vi "PH_Tektronix_7000.get Channel Configuration.vi"(0 "i ref in":refnum<vi>, 1 "Channel":u16(ring) items=["Channel 1", "Channel 2", "Channel 3", "Channel 4", "Math 1", "Math 2", "Math 3", "Math 4", "Reference 1", "Reference 2", "Reference 3", "Reference 4"], 5 "error IO":errorcluster) -> (14 "i ref out":refnum<vi>, 19 "error out":errorcluster)   [LabVIEW 2014, in "PH_Tektronix_7000.lvlib"]
doc: "If the connection is established, the current channel configuration is queried and written to own attributes as well as the errors."
uses:
  PH_Tektronix_7000.lvlib
  PH_Tektronix_7000.Channel Config.ctl
  instr.lib/Tektronix7000Series/Tektronix 7000 Series - Driver np.lvlib
panel:
  in  "CH cluster":T1={"Enable Channel"=FALSE, "Bandwidth"=0, "Input Impedance"=0, "Vertical Coupling"=1, "Probe Attenuation"=1.0, "Range [V/div]"=10.0, "Position [div]"=0.0, "Bandwidth raw"=""} {"Vertical Coupling" items=["AC", "DC", "Ground"]; "Input Impedance" items=["1M", "50"]; "Bandwidth" items=["FULL", "500 MHz", "250 MHz", "150 MHz", "20 MHz"]}
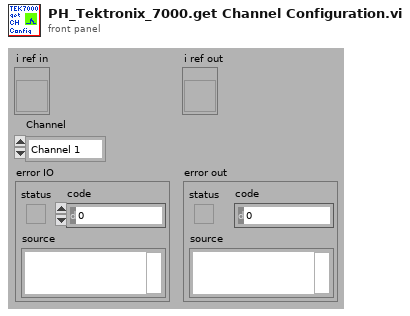
[diagram p1: front panel]
types:
  T1 = typedef "PH_Tektronix_7000.lvlib/PH_Tektronix_7000.Channel Config.ctl" = cluster{"Enable Channel":bool, "Bandwidth":u16, "Input Impedance":u16, "Vertical Coupling":u16, "Probe Attenuation":dbl, "Range [V/div]":dbl, "Position [div]":dbl, "Bandwidth raw":string}
  T2 = typedef "PH_Tektronix_7000.lvlib/PH_Tektronix_7000.i attribute.ctl" = cluster{"VISA Resource Name":refnum<visa-resource-name>, "IDN":cluster{"Instrument Driver":string, "Instrument Firmware":string, "Model":string, "Serial Number":string}, "Selftest":cluster{"Result":i32, "Message":string}, "Trigger Configuration":T3, "Acquisition Configuration":T4, "GUI Refs":T5, "State":T6, "Error Message":string, "Allow Prdc Loop?":bool, "Channel 1":T1, "Channel 2":T1, "Channel 3":T1, "Channel 4":T1, "Data CH 1":waveform(dbl), "Data CH 2":waveform(dbl), "Data CH 3":waveform(dbl), "Data CH 4":waveform(dbl), "Allow config?":bool, "Name Channel 1":string, "Name Channel 2":string, "Name Channel 3":string, "Name Channel 4":string, "Fetch Data before sending to PSDB?":bool, "Constructor passed?":bool, "Data taken at":timestamp, "Plot Colors":u32[], "Default VISA Resource":string}
  T3 = typedef "PH_Tektronix_7000.lvlib/PH_Tektronix_7000.Trigger Config.ctl" = cluster{"Source":u16, "Level [V]":dbl, "Slope":u16, "Coupling":u16, "Trigger Mode":u16}
  T4 = typedef "PH_Tektronix_7000.lvlib/PH_Tektronix_7000.Acquisition Config.ctl" = cluster{"Record Length":u32, "Timebase [s/div]":dbl, "Position [%]":dbl, "Acquisition Type":u16, "Average Waveforms":i32, "Envelope Waveforms":i32, "WfmDB Samples":i32, "Continuous?":bool, "Delay [s]":dbl, "Run?":bool}
  T5 = typedef "PH_Tektronix_7000.lvlib/PH_Tektronix_7000.GUI Refs.ctl" = cluster{"Graph":refnum<vi>, "State":refnum<vi>, "Delete":refnum<vi>, "VISA Resource":refnum<vi>, "Allow Configure":refnum<vi>, "Fetch Data":refnum<vi>, "Fetch before sending Data to PSDB":refnum<vi>, "Name Channel 1":refnum<vi>, "Name Channel 2":refnum<vi>, "Name Channel 3":refnum<vi>, "Name Channel 4":refnum<vi>, "Prdc Intervall [ms]":refnum<vi>, "Data taken":refnum<vi>, "Model":refnum<vi>, "Serial Number":refnum<vi>, "Firmware":refnum<vi>, "Driver":refnum<vi>, "Acquisition":refnum<vi>, "Trigger":refnum<vi>, "Cursor: D Time [s]":refnum<vi>, "Cursor: D Signal [V]":refnum<vi>, "Channel 1":refnum<vi>, "Channel 2":refnum<vi>, "Channel 3":refnum<vi>, "Channel 4":refnum<vi>}
  T6 = typedef "PH_StatusHandler.lvlib/PH_StatusHandler.Status.ctl" = i16
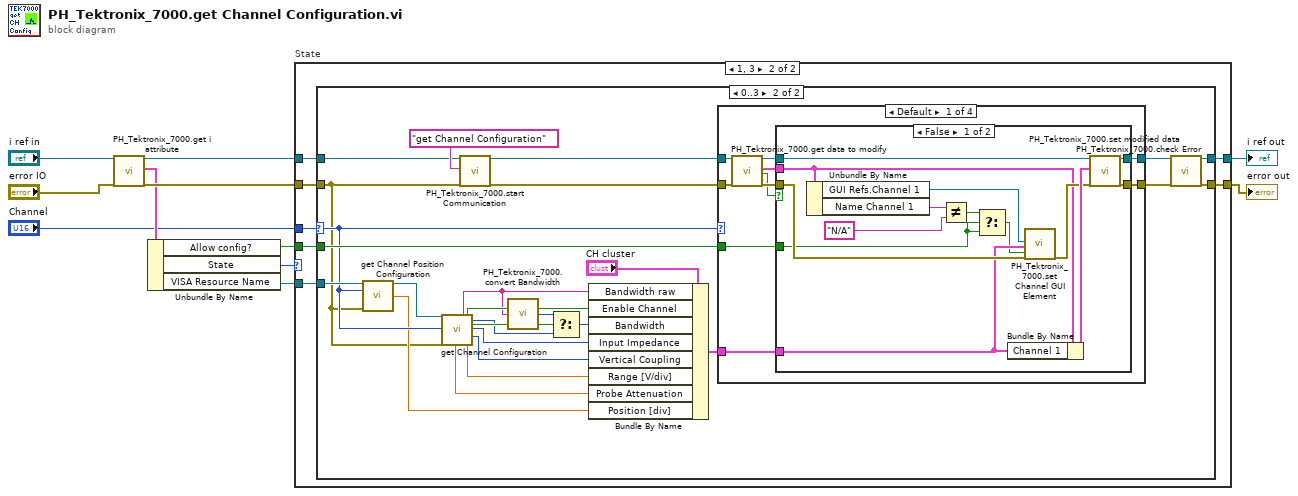
[diagram p0: block diagram]
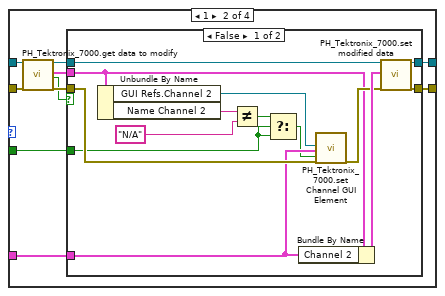
[diagram p5: hidden frame]
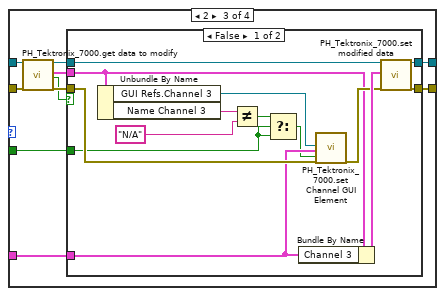
[diagram p7: hidden frame]
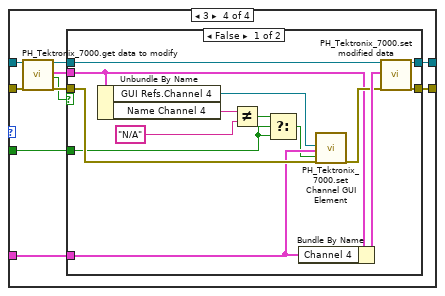
[diagram p9: hidden frame]
diagram:
  n1 = call "PH_Tektronix_7000.get i attribute.vi"("i ref in"="i ref in", "error in (no error)"="error IO") -> ("i ref out"=w7:refnum<vi>, "i attribute"=w9:T2, "error out"=w10:errorcluster)  [unwired: 15 in]
  n2 = Unbundle By Name(w9) -> ("Allow config?"=w3:bool, "State"=w2:T6, "VISA Resource Name"=w1:refnum<visa-resource-name>)
  n3 = case "State" shown="1, 3" w2 {
    tunnel: [w13 w20] -> w11
    tunnel: w10 -> [w12 w19]
    tunnel: w1 -> [_ w18]
    tunnel: w7 -> [w13 w17]
    tunnel: [w12 w16] -> w5
    tunnel: w3 -> [_ w15]
    tunnel: "Channel" -> [_ w14]
    frame Default {
    }
    frame 1, 3 {
      n4 = case shown="0..3" w14 {
        selector: w14 -> [_ w25]
        tunnel: [w22 w48] -> w20
        tunnel: w19 -> [w21 w23]
        tunnel: w18 -> [_ w38]
        tunnel: w17 -> [w22 w43]
        tunnel: [w21 w46] -> w16
        tunnel: w15 -> [_ w33]
        frame Default {
        }
        frame 0..3 {
          n5 = call "get Channel Position Configuration.vi"("VISA resource name"=w38, "Channel (0: Channel 1)"=w25, "error in (no error)"=w23) -> ("VISA resource name out"=w26:refnum<visa-resource-name>, "Vertical Position [div]"=w24:dbl)  [unwired: 10 in, 1 out]
          n6 = call "get Channel Configuration.vi"("VISA resource name"=w26, "Channel (0: Channel 1)"=w25, "error in (no error)"=w23) -> ("Probe Attenuation"=w34:dbl, "Bandwidth raw"=w28:string, "Channel enabled?"=w29:bool, "Vertical Range [V]"=w35:dbl, "Bandwidth"=w31:u16, "Bandwidth not found"=w32:bool, "Input Impedance"=w37:u16, "Vertical Coupling"=w36:u16)  [unwired: 11 in, 6 out]
          n7 = call "PH_Tektronix_7000.start Communication.vi"("i ref in"=w43, "Action"="get Channel Configuration", "error in"=w23) -> ("i ref out"=w42:refnum<vi>, "error out"=w41:errorcluster)  [unwired: 15 in]
          n8 = call "PH_Tektronix_7000.convert Bandwidth.vi"("Bandwidth raw"=w28) -> ("Bandwidth"=w27:u16)
          n9 = Select(t=w27, s=w32, f=w31) -> (s? t:f=w30:u16)
          n10 = Bundle By Name(cluster="CH cluster", "Bandwidth raw"=w28, "Enable Channel"=w29, "Bandwidth"=w30, "Input Impedance"=w37, "Vertical Coupling"=w36, "Range [V/div]"=w35, "Probe Attenuation"=w34, "Position [div]"=w24) -> (w39:T1)
          n11 = case "Channel Label" shown="Default" w25 {
            tunnel: [w54 w80 w106 w132] -> w47
            tunnel: w41 -> [w51 w77 w103 w129]
            tunnel: w42 -> [w52 w78 w104 w130]
            tunnel: [w53 w79 w105 w131] -> w45
            tunnel: w39 -> [w50 w76 w102 w128]
            tunnel: w33 -> [w49 w75 w101 w127]
            frame Default {
              n12 = call "PH_Tektronix_7000.get data to modify.vi"("i ref in"=w52, "error in (no error)"=w51) -> ("i ref out"=w57:refnum<vi>, "i attribute"=w55:T2, "timed out"=w56:bool, "error out"=w58:errorcluster)  [unwired: 14 in]
              n13 = case shown="False" w56 {
                tunnel: [w69 w73] -> w53
                tunnel: w58 -> [w68 w73]
                tunnel: w57 -> [w72 w74]
                tunnel: [w70 w74] -> w54
                tunnel: w55 -> [w66 _]
                tunnel: w50 -> [w65 _]
                tunnel: w49 -> [w63 _]
                frame False {
                  n14 = Unbundle By Name(w66) -> ("GUI Refs.Channel 1"=w59:refnum<vi>, "Name Channel 1"=w62:string)
                  n15 = Not Equal?(x=w62, y="N/A") -> (x != y?=w60:bool)
                  n16 = Select(t=w60, s=w63, f=w63) -> (s? t:f=w64:bool)
                  n17 = Bundle By Name(cluster=w66, "Channel 1"=w65) -> (w71:T2)
                  n18 = call "PH_Tektronix_7000.set Channel GUI Element.vi"("GUI Ref Channel"=w59, "Channel Config"=w65, "enabled?"=w64, "error in"=w68) -> ("error out"=w67:errorcluster)  [unwired: 15 in]
                  n19 = call "PH_Tektronix_7000.set modified data.vi"("i ref in"=w72, "i attribute"=w71, "error in (no error)"=w67) -> ("i ref out"=w70:refnum<vi>, "error out"=w69:errorcluster)  [unwired: 15 in]
                }
                frame True {
                }
              }
            }
            frame 1 {
              n20 = call "PH_Tektronix_7000.get data to modify.vi"("i ref in"=w78, "error in (no error)"=w77) -> ("i ref out"=w83:refnum<vi>, "i attribute"=w81:T2, "timed out"=w82:bool, "error out"=w84:errorcluster)  [unwired: 14 in]
              n21 = case shown="False" w82 {
                tunnel: [w95 w99] -> w79
                tunnel: w84 -> [w94 w99]
                tunnel: w83 -> [w98 w100]
                tunnel: [w96 w100] -> w80
                tunnel: w81 -> [w92 _]
                tunnel: w76 -> [w90 _]
                tunnel: w75 -> [w88 _]
                frame False {
                  n22 = Unbundle By Name(w92) -> ("GUI Refs.Channel 2"=w91:refnum<vi>, "Name Channel 2"=w87:string)
                  n23 = Not Equal?(x=w87, y="N/A") -> (x != y?=w85:bool)
                  n24 = Select(t=w85, s=w88, f=w88) -> (s? t:f=w89:bool)
                  n25 = Bundle By Name(cluster=w92, "Channel 2"=w90) -> (w97:T2)
                  n26 = call "PH_Tektronix_7000.set Channel GUI Element.vi"("GUI Ref Channel"=w91, "Channel Config"=w90, "enabled?"=w89, "error in"=w94) -> ("error out"=w93:errorcluster)  [unwired: 15 in]
                  n27 = call "PH_Tektronix_7000.set modified data.vi"("i ref in"=w98, "i attribute"=w97, "error in (no error)"=w93) -> ("i ref out"=w96:refnum<vi>, "error out"=w95:errorcluster)  [unwired: 15 in]
                }
                frame True {
                }
              }
            }
            frame 2 {
              n28 = call "PH_Tektronix_7000.get data to modify.vi"("i ref in"=w104, "error in (no error)"=w103) -> ("i ref out"=w109:refnum<vi>, "i attribute"=w107:T2, "timed out"=w108:bool, "error out"=w110:errorcluster)  [unwired: 14 in]
              n29 = case shown="False" w108 {
                tunnel: [w121 w125] -> w105
                tunnel: w110 -> [w120 w125]
                tunnel: w109 -> [w124 w126]
                tunnel: [w122 w126] -> w106
                tunnel: w107 -> [w118 _]
                tunnel: w102 -> [w116 _]
                tunnel: w101 -> [w114 _]
                frame False {
                  n30 = Unbundle By Name(w118) -> ("GUI Refs.Channel 3"=w117:refnum<vi>, "Name Channel 3"=w113:string)
                  n31 = Not Equal?(x=w113, y="N/A") -> (x != y?=w111:bool)
                  n32 = Select(t=w111, s=w114, f=w114) -> (s? t:f=w115:bool)
                  n33 = Bundle By Name(cluster=w118, "Channel 3"=w116) -> (w123:T2)
                  n34 = call "PH_Tektronix_7000.set Channel GUI Element.vi"("GUI Ref Channel"=w117, "Channel Config"=w116, "enabled?"=w115, "error in"=w120) -> ("error out"=w119:errorcluster)  [unwired: 15 in]
                  n35 = call "PH_Tektronix_7000.set modified data.vi"("i ref in"=w124, "i attribute"=w123, "error in (no error)"=w119) -> ("i ref out"=w122:refnum<vi>, "error out"=w121:errorcluster)  [unwired: 15 in]
                }
                frame True {
                }
              }
            }
            frame 3 {
              n36 = call "PH_Tektronix_7000.get data to modify.vi"("i ref in"=w130, "error in (no error)"=w129) -> ("i ref out"=w135:refnum<vi>, "i attribute"=w133:T2, "timed out"=w134:bool, "error out"=w136:errorcluster)  [unwired: 14 in]
              n37 = case shown="False" w134 {
                tunnel: [w147 w151] -> w131
                tunnel: w136 -> [w146 w151]
                tunnel: w135 -> [w150 w152]
                tunnel: [w148 w152] -> w132
                tunnel: w133 -> [w144 _]
                tunnel: w128 -> [w142 _]
                tunnel: w127 -> [w140 _]
                frame False {
                  n38 = Unbundle By Name(w144) -> ("GUI Refs.Channel 4"=w143:refnum<vi>, "Name Channel 4"=w139:string)
                  n39 = Not Equal?(x=w139, y="N/A") -> (x != y?=w137:bool)
                  n40 = Select(t=w137, s=w140, f=w140) -> (s? t:f=w141:bool)
                  n41 = Bundle By Name(cluster=w144, "Channel 4"=w142) -> (w149:T2)
                  n42 = call "PH_Tektronix_7000.set Channel GUI Element.vi"("GUI Ref Channel"=w143, "Channel Config"=w142, "enabled?"=w141, "error in"=w146) -> ("error out"=w145:errorcluster)  [unwired: 15 in]
                  n43 = call "PH_Tektronix_7000.set modified data.vi"("i ref in"=w150, "i attribute"=w149, "error in (no error)"=w145) -> ("i ref out"=w148:refnum<vi>, "error out"=w147:errorcluster)  [unwired: 15 in]
                }
                frame True {
                }
              }
            }
          }
          n44 = call "PH_Tektronix_7000.check Error.vi"("i ref in"=w47, "error in"=w45) -> ("i ref out"=w48:refnum<vi>, "error out"=w46:errorcluster)  [unwired: 16 in]
        }
      }
    }
  }
  "i ref out" <- w11
  "error out" <- w5
